vi "Untitled 3.vi"   [LabVIEW 2020]
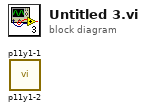
[diagram p0: block diagram]
diagram:
  n1 = call "p11y1-2.vi"() -> ()  [unwired: 12 in]
  n2 = call "p11y1-1.vi"() -> ()  [unwired: 12 in]
